vi "HostPacket.vi"(11 "Parameters":T1) -> (2 "string":string, 3 "Byte Array":u8[](array[numeric]) format="%x")   [LabVIEW 2014]
uses:
  Parameters.ctl
  PID Mode.ctl
  InputSimulationMode.ctl
panel:
  # "0xb6 0xf3 0x9d 0x3f"
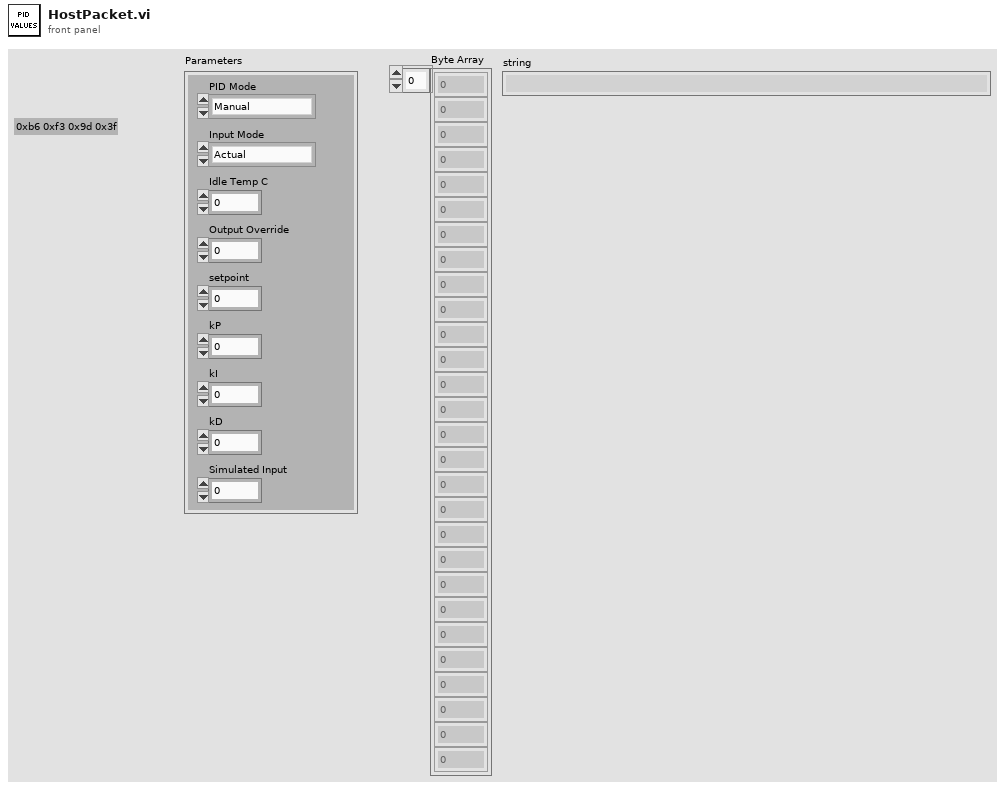
[diagram p1: front panel]
types:
  T1 = typedef "Parameters.ctl" = cluster{"PID Mode":T2, "Input Mode":T3, "Idle Temp C":i16, "Output Override":i16, "setpoint":sgl, "kP":sgl, "kI":sgl, "kD":sgl, "Simulated Input":sgl}
  T2 = typedef "PID Mode.ctl" = enum8{"Manual", "Automatic"}
  T3 = typedef "InputSimulationMode.ctl" = enum8{"Actual", "Simulated"}
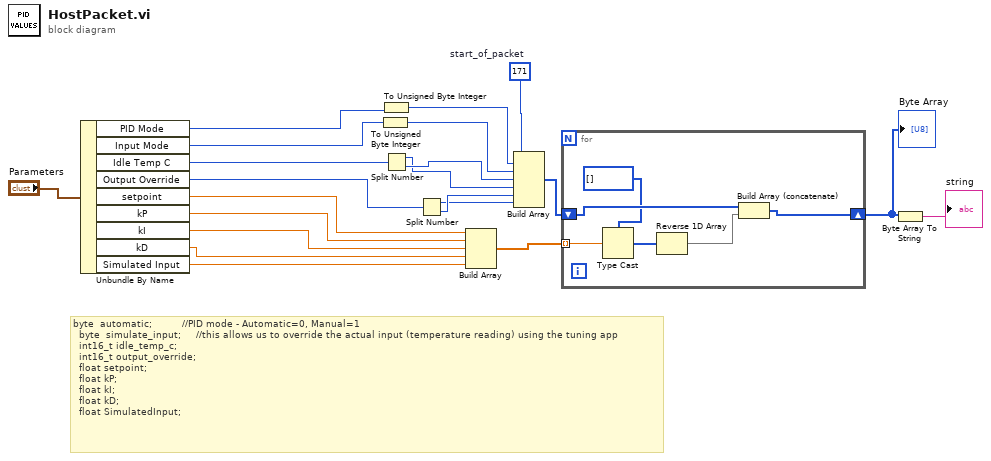
[diagram p0: block diagram]
diagram:
  w16 = u8 171  # start_of_packet
  # "byte  automatic;          //PID mode - Automatic=0, Manual=1\n  byte  simulate_input;     //this allows us to override the actual input (temperature reading) using the tuning app\n  int16_t idle_temp_c;\n  int16_t output_override;\n  float setpoint;\n  float kP;\n  float kI;\n  float kD;\n  float SimulatedInput;"
  n1 = Unbundle By Name("Parameters") -> ("PID Mode"=w14:T2, "Input Mode"=w13:T3, "Idle Temp C"=w8:i16, "Output Override"=w5:i16, "setpoint"=w6:sgl, "kP"=w12:sgl, "kI"=w11:sgl, "kD"=w10:sgl, "Simulated Input"=w9:sgl)
  n2 = To Unsigned Byte Integer(number=w13) -> (unsigned 8bit integer=w18:u8)
  n3 = To Unsigned Byte Integer(number=w14) -> (unsigned 8bit integer=w19:u8)
  n4 = Split Number(x=w8) -> (hi(x)=w3:u8, lo(x)=w4:u8)
  n5 = Split Number(x=w5) -> (hi(x)=w1:u8, lo(x)=w2:u8)
  n6 = Build Array(w6, w12, w11, w10, w9) -> (w20:sgl[])
  n7 = Build Array(w16, w19, w18, w4, w3, w2, w1) -> (w17:u8[])
  n8 = for {
    tunnel: w20 -> [w27] mode=indexing
    shift-right: [w22] -> w7
    shift-left: w17 -> [w26]
    n9 = Type Cast(type=u8[] [], x=w27) -> (*(type *) &x=w24:u8[])
    n10 = Reverse 1D Array(array=w24) -> (reversed array=w23:u8[])
    n11 = Build Array (concatenate)(w26, w23) -> (w22:u8[])
  }
  "Byte Array" <- w7
  n12 = Byte Array To String(unsigned byte array=w7) -> (string=→"string":string)
